vi "DI Read Line.vi"(7 "State":u16, 8 "error in (no error)":errorcluster caption="错误输入（无错误）", 9 "Line":u16, 10 "Port":u16, 11 "CardNumber":u16) -> (0 "error out":errorcluster caption="错误输出", 3 "function return":i16, 5 "State out":u16)   [LabVIEW 2017, in "Adlink IO.lvlib"]
doc: "I16 __stdcall DI_ReadLine(U16 CardNumber, U16 Port, U16 Line, U16 *State);"
uses:
  Adlink IO.lvlib
  PCI-Dask.dll
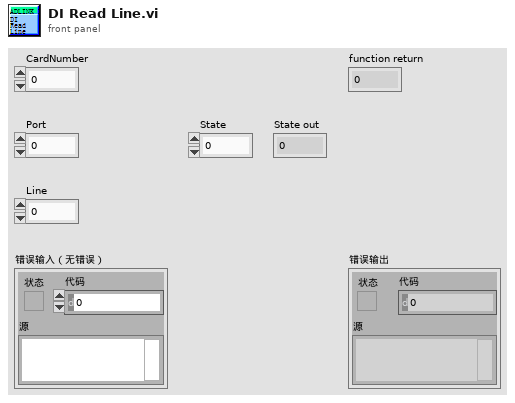
[diagram p1: front panel]
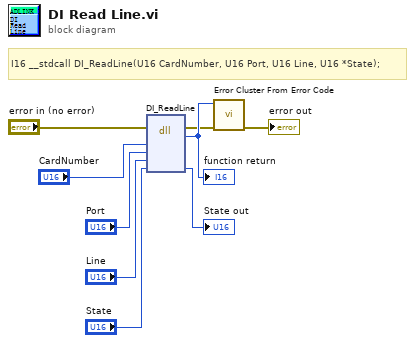
[diagram p0: block diagram]
diagram:
  # "I16 __stdcall DI_ReadLine(U16 CardNumber, U16 Port, U16 Line, U16 *State);"
  n1 = dll-call lib="D:/Program/Dyson X692 UI Provison Tester V1.0.0/HardWare/ADLINK/IO/Adlink IO/PCI-Dask.*" fn="DI_ReadLine"(error in="error in (no error)", "CardNumber"="CardNumber", "Port"="Port", "Line"="Line", "State"="State") -> (error out=w2:errorcluster, w9:i16, "State"=→"State out":u16)  [unwired: 5 in, 1 out]
  "function return" <- w9
  n2 = call <vilib>:"Error Cluster From Error Code.vi"("error in (no error)"=w2, "error code (0)"=w9) -> ("error out"=→"error out":errorcluster)  [unwired: 7 in]
